vi "Take fron panel screenshot.vi"(4 "error in (no error)":errorcluster, 5 "VI path":path=path "E:/Tenor/LabVIEW/labview_testcases/tenor/pll/ldo_psrr/Labview pulse psrr capture and process.vi", 6 "Image path":path, 7 "Visible area only? (f)":bool, 8 "File type (.jpg)":enum16{".bmp", ".png", ".jpg"}(ring)=enum.".jpg") -> (0 "error out":errorcluster)   [LabVIEW 2021]
doc: "This example captures an image of the front panel of a VI and saves the image to a JPG, PNG, or BMP file."
panel:
  out "Image path":path
  # "Select Help»Show Context Help and move the cursor over the VI icon to display help for this VI."
  # "1. Select the file type for the image you want to save.\n2. Specify the path where you want to save image file.\n3. Specify the path to the VI whose front panel you want to take a screenshot of.\n4. Run the VI."
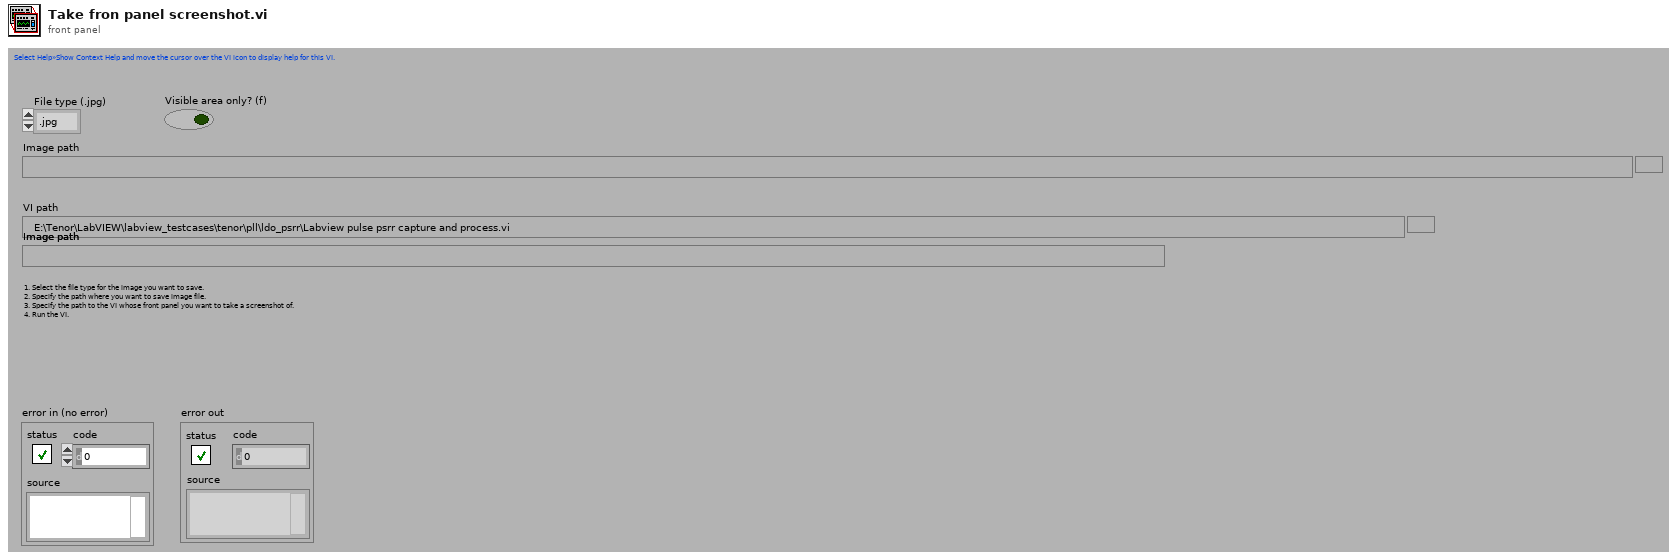
[diagram p1: front panel]
types:
  T1 = typedef "imagedata.ctl" = cluster{"image type":i32, "image depth":i32, "image":u8[], "mask":u8[], "colors":u32[], "Rectangle":cluster{"left":i16, "top":i16, "right":i16, "bottom":i16}}
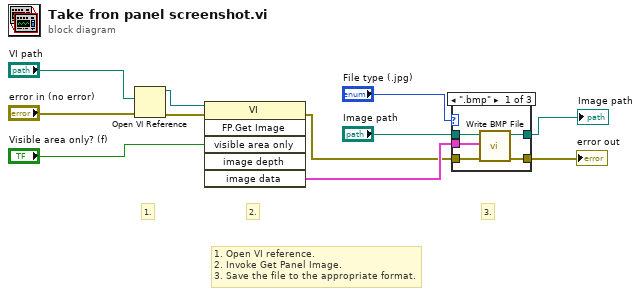
[diagram p0: block diagram]
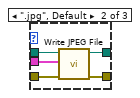
[diagram p2: hidden frame]
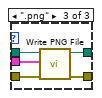
[diagram p3: hidden frame]
diagram:
  # "1. Open VI reference.\n2. Invoke Get Panel Image.\n3. Save the file to the appropriate format."
  # "3."
  # "2."
  # "1."
  n1 = Open VI Reference(vi path="VI path", error in (no error)="error in (no error)") -> (vi reference=w11:refnum<vi>, error out=w8:errorcluster)  [unwired: 4 in]
  n2 = invoke class="VI" method="FP.Get Image"(reference=w11, error in=w8, "visible area only"="Visible area only? (f)") -> (error out=w7:errorcluster, "image data"=w9:T1)  [unwired: 3 in, 4 out]
  n3 = case shown="\".bmp\"" "File type (.jpg)" {
    tunnel: w9 -> [w15 w20 w25]
    tunnel: w7 -> [w14 w21 w26]
    tunnel: "Image path" -> [w16 w19 w24]
    tunnel: [w13 w18 w23] -> w2
    tunnel: [w12 w17 w22] -> w1
    frame ".bmp" {
      n4 = call <vilib>:"Write BMP File.vi"("error in (no error)"=w14, "image data"=w15, "path to BMP file"=w16) -> ("error out"=w13:errorcluster, "path"=w12:path)  [unwired: 7 in]
    }
    frame ".jpg", Default {
      n5 = call <vilib>:"Write JPEG File.vi"("error in (no error)"=w21, "image data"=w20, "path to JPEG file"=w19) -> ("error out"=w18:errorcluster, "path"=w17:path)  [unwired: 7 in]
    }
    frame ".png" {
      n6 = call <vilib>:"Write PNG File.vi"("error in (no error)"=w26, "image data"=w25, "path to PNG file"=w24) -> ("error out"=w23:errorcluster, "path"=w22:path)  [unwired: 7 in]
    }
  }
  "error out" <- w2
  "Image path" <- w1
